vi "Go to to field (stable).vi"(8 "error in":errorcluster, 10 "Desired field":dbl[unit], 11 "varian in":refnum<class "Varian Magnet.lvclass">) -> (0 "error out":errorcluster, 1 "Current control voltage":dbl, 2 "Current field":dbl[unit], 3 "varian out":refnum<class "Varian Magnet.lvclass">)   [LabVIEW 2009, in "Varian Magnet.lvclass"]
uses:
  Varian Magnet.lvclass
  Varian Magnet.lvclass/Varian Magnet.ctl
  <vilib>/DAQmx/create/channels.llb/DAQmx Create Channel (AO-Voltage-Basic).vi
  Varian Max Field.vi
panel:
  out "Waveform Chart":dbl[unit](graph)
  out "Time elapsed":dbl
  # "VOLTAGE KNOB SETTINGS:\n\nMAIN SETTING:\n40 V on High Voltage Knob\n\nFor fields 0.1 T increasing  0.45 T\n fast response and all decreasing fields\nP= -350\nI= -12\nD= 1\n\nFor fields 0.5 T increasing to 0.9 T\nuse PID gains with smallest peak and \nfastest response\nP= -75\nI= -0.5\nD= -1\n\nDO NOT GO ABOVE 0.9 T\n\n\n30 V SETTING:\nBest for fields below 0.5 T. 0.5 MAX comfortable range. Faster with fields below 0.1 T than on the 40 V setting.\nP= -110\nI= -2\nD= 1\n\n50 V SETTING:\nNot reliable"
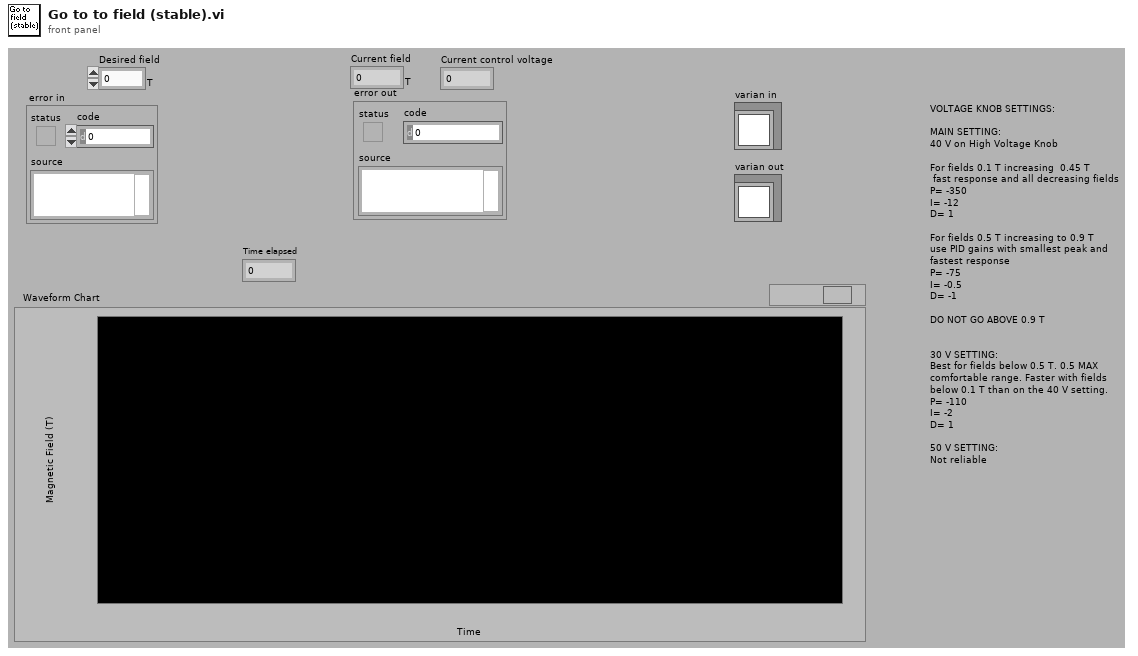
[diagram p1: front panel]
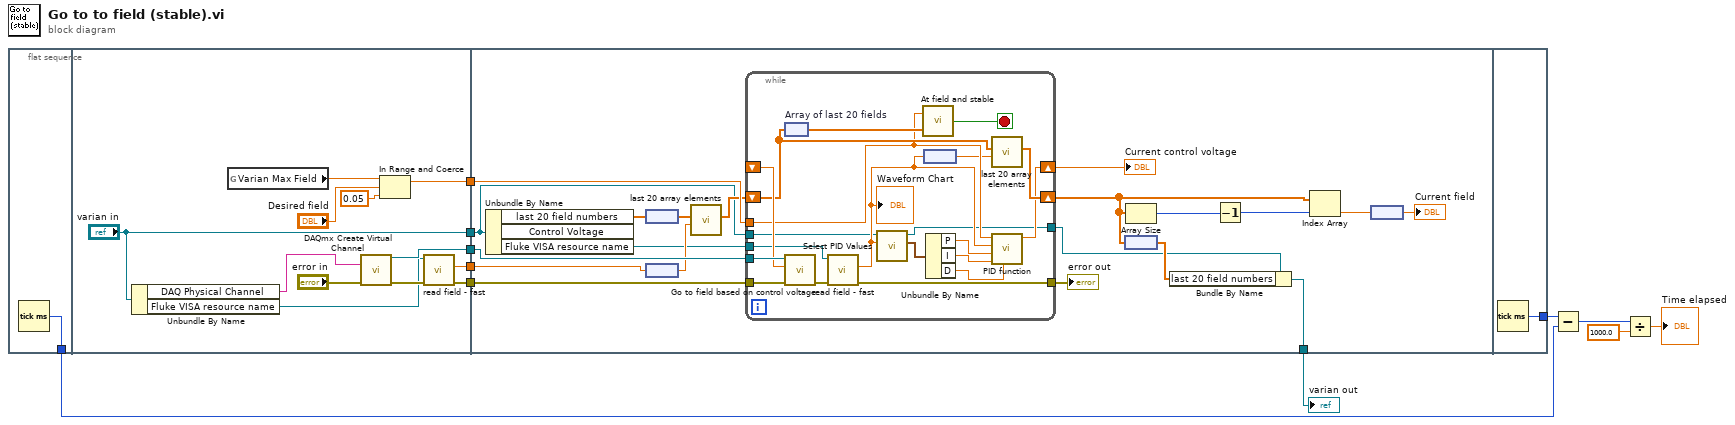
[diagram p0: block diagram]
diagram:
  n1 = flat-sequence {
    tunnel: [w12] -> w8
    tunnel: [w21] -> w6
    tunnel: [w18] -> w5
    tunnel: [w17] -> w4
    tunnel: [w16] -> w3
    tunnel: ["varian in"] -> w1
    tunnel: w6 -> [w38]
    tunnel: w5 -> [w37]
    tunnel: w4 -> [w36]
    tunnel: w3 -> [w35]
    tunnel: [w34] -> w2
    tunnel: w1 -> [w26]
    tunnel: [w65] -> w9
    frame #0 {
      n2 = Tick Count (ms)() -> (millisecond timer value=w12:u32)
    }
    frame #1 {
      n3 = Unbundle By Name("varian in") -> ("DAQ Physical Channel"=w14:tag, "Fluke VISA resource name"=w15:refnum<visa-resource-name>)
      n4 = global read "Varian Max Field.vi" "Varian Max Field"() -> (w23:dbl[unit])
      n5 = call-poly <vilib>:"DAQmx Create Virtual Channel.vi"("physical channels"=w14, "error in"="error in") -> ("task out"=w16:refnum<k21>, "error out"=w20:errorcluster)  [unwired: 7 in, 5 out]
      n6 = In Range and Coerce(upper limit=w23, x="Desired field", lower limit=dbl[unit] 0.05) -> (coerced(x)=w21:dbl[unit])  [unwired: 1 out]
      n7 = call "read field - fast.vi"("error in (no error)"=w20, "VISA resource name"=w15) -> ("error out"=w18:errorcluster, "Current field (T)"=w17:dbl[unit])  [unwired: 8 out]
    }
    frame #2 {
      n8 = Unbundle By Name(w26) -> ("last 20 field numbers"=w29:dbl[unit][], "Fluke VISA resource name"=w27:refnum<visa-resource-name>)  [unwired: 1 out]
      n9 = node(w29) -> (w28:dbl[])
      n10 = node(w36) -> (w31:dbl)
      n11 = call "last 20 array elements.vi"("number to be inserted at end"=w31, "input array"=w28) -> ("output array"=w30:dbl[])  [unwired: 9 out]
      n12 = while {
        tunnel: w35 -> [w64]
        shift-right: [w60] -> w40
        shift-left: _ -> [w63]
        tunnel: w38 -> [w58]
        shift-right: [w62] -> w33
        shift-left: w30 -> [w61]
        tunnel: w37 -> [w57]
        tunnel: [w55] -> w41
        tunnel: w27 -> [w47]
        tunnel: w26 -> [w46]
        tunnel: [w45] -> w25
        stop <- w48 stop-if-true
        n13 = node "Array of last 20 fields"(w61) -> (w59:dbl[unit][])
        n14 = call "Go to field based on control voltage.vi"("error in"=w57, "Control Voltage"=w63, "task in"=w64) -> ("error out"=w56:errorcluster)  [unwired: 8 out]
        n15 = call "read field - fast.vi"("error in (no error)"=w56, "VISA resource name"=w47) -> ("error out"=w55:errorcluster, "Current field (T)"=w49:dbl[unit])  [unwired: 8 out]
        "Waveform Chart" <- w49
        n16 = call "Select PID Values.vi"("current field"=w49, "varian in"=w46) -> ("PID output"=w53:cluster{"I":dbl, "D":dbl, "P":dbl}, "varian out"=w45:refnum<class "Varian Magnet.lvclass">)  [unwired: 8 in]
        n17 = call "At field and stable.vi"("last 20 field numbers"=w59, "Desired field"=w58) -> ("At field and stable?"=w48:bool)
        n18 = node(w49) -> (w54:dbl)
        n19 = Unbundle By Name(w53) -> ("P"=w52:dbl, "I"=w51:dbl, "D"=w50:dbl)
        n20 = call "last 20 array elements.vi"("number to be inserted at end"=w54, "input array"=w61) -> ("output array"=w62:dbl[])  [unwired: 9 out]
        n21 = call "PID function.vi"("D"=w50, "I"=w51, "P"=w52, "Current Field"=w49, "Field Desired"=w58) -> ("Numeric"=w60:dbl)  [unwired: 6 out]
      }
      "error out" <- w41
      "Current control voltage" <- w40
      n22 = node(w33) -> (w32:dbl[unit][])
      n23 = Array Size(array=w33) -> (size(s)=w44:i32)
      n24 = Bundle By Name(cluster=w25, "last 20 field numbers"=w32) -> (w34:refnum<class "Varian Magnet.lvclass">)
      n25 = Decrement(x=w44) -> (x-1=w43:i32)
      n26 = Index Array(array=w33, index=w43) -> (element=w42:dbl)
      n27 = node(w42) -> (→"Current field":dbl[unit])
    }
    frame #3 {
      n28 = Tick Count (ms)() -> (millisecond timer value=w65:u32)
    }
  }
  n29 = Subtract(x=w9, y=w8) -> (x-y=w11:u32)
  n30 = Divide(x=w11, y=1000.0) -> (x/y=→"Time elapsed":dbl)
  "varian out" <- w2
